vi "startTcpServer.vi"(8 "error in (no error)":errorcluster) -> (0 "error out":errorcluster, 2 "TcpServer out":refnum<class "TcpServer.lvclass">, 3 "UserEvents":T1)   [LabVIEW 2018]
doc: "Start the TCP server."
uses:
  src/TcpServer/TcpServer.lvclass
  src/TcpServerBase/typedef/connStatusCluster.ctl
  src/TcpServer/configServerTypeDef.ctl
  src/TcpServerTel/typedef/enqueueOptionsTypeDef.ctl
  src/FactoryTcpServer/FactoryTcpServer.lvclass
  src/TcpServer/runServer.vi
  src/TcpServerTel/TcpServerTel.lvclass
  src/TcpServerBase/TcpServerBase.lvclass
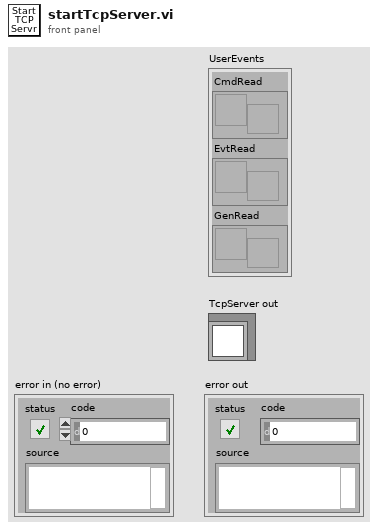
[diagram p1: front panel]
types:
  T1 = cluster{"CmdRead":refnum<user-event>, "EvtRead":refnum<user-event>, "GenRead":refnum<user-event>}
  T2 = typedef "TcpServer.lvclass/configServerTypeDef.ctl" = cluster{"cmdServerPort":u16, "telServerPort":u16, "timeoutServerInMs":i32, "serverBytesToRead":i32, "maxSizeQueueTcpClientFromDds":i32, "EnqueueOptions":T3, "timeoutQueueTcpClientFromDds (ms)":i32, "maxSizeQueueTcpClient":i32, "timeoutInMs":i32}
  T3 = typedef "TcpServerTel.lvclass/enqueueOptionsTypeDef.ctl" = enum16{"lossy enqueue", "normal enqueue"}
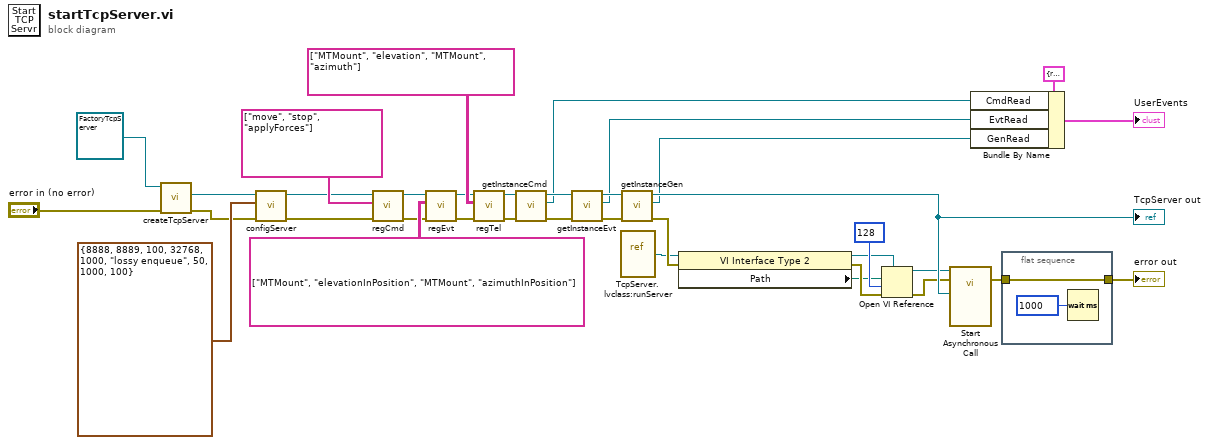
[diagram p0: block diagram]
diagram:
  n1 = call "createTcpServer.vi"("error in (no error)"="error in (no error)", "FactoryTcpServer in"=refnum<class "FactoryTcpServer.lvclass"> refnum) -> ("error out"=w3:errorcluster, "TcpServer out"=w4:refnum<class "TcpServer.lvclass">)  [unwired: 7 in, 1 out]
  n2 = call "configServer.vi"("error in (no error)"=w3, "ServerConfiguration"=T2 {"cmdServerPort"=8888, "telServerPort"=8889, "timeoutServerInMs"=100, "serverBytesToRead"=32768, "maxSizeQueueTcpClientFromDds"=1000, "EnqueueOptions"=enum."lossy enqueue", "timeoutQueueTcpClientFromDds (ms)"=50, "maxSizeQueueTcpClient"=1000, "timeoutInMs"=100}, "tcpServer in"=w4) -> ("error out"=w32:errorcluster, "tcpServer out"=w13:refnum<class "TcpServer.lvclass">)  [unwired: 7 in]
  n3 = call "regCmd.vi"("error in (no error)"=w32, "cmdReg"=string[] ["move", "stop", "applyForces"], "tcpServer in"=w13) -> ("error out"=w12:errorcluster, "tcpServer out"=w25:refnum<class "TcpServer.lvclass">)  [unwired: 7 in]
  n4 = call "regEvt.vi"("error in (no error)"=w12, "evtReg"=string[][] [["MTMount", "elevationInPosition"], ["MTMount", "azimuthInPosition"]], "tcpServer in"=w25) -> ("error out"=w24:errorcluster, "tcpServer out"=w29:refnum<class "TcpServer.lvclass">)  [unwired: 7 in]
  n5 = call "regTel.vi"("error in (no error)"=w24, "telReg"=string[][] [["MTMount", "elevation"], ["MTMount", "azimuth"]] ("regTel"), "tcpServer in"=w29) -> ("error out"=w28:errorcluster, "tcpServer out"=w30:refnum<class "TcpServer.lvclass">)  [unwired: 7 in]
  n6 = call "getInstanceCmd.vi"("error in (no error)"=w28, "tcpServer in"=w30) -> ("error out"=w14:errorcluster, "CmdRead"=w10:refnum<user-event>, "tcpServer out"=w16:refnum<class "TcpServer.lvclass">)  [unwired: 7 in]
  n7 = call "getInstanceEvt.vi"("error in (no error)"=w14, "tcpServer in"=w16) -> ("error out"=w15:errorcluster, "EvtRead"=w9:refnum<user-event>, "tcpServer out"=w27:refnum<class "TcpServer.lvclass">)  [unwired: 7 in]
  n8 = vi-ref "TcpServer.lvclass:runServer.vi"() -> (w17:refnum<vi>)
  n9 = call "getInstanceGen.vi"("error in (no error)"=w15, "tcpServer in"=w27) -> ("error out"=w26:errorcluster, "GenRead"=w8:refnum<user-event>, "tcpServer out"=w36:refnum<class "TcpServer.lvclass">)  [unwired: 7 in]
  "TcpServer out" <- w36
  n10 = property class="VI Interface Type 2"(reference=w17, error in=w26) -> (reference out=w19:refnum<vi>, error out=w22:errorcluster, "Path"=w18:path)
  n11 = Open VI Reference(type specifier VI Refnum (for type only)=w19, vi path=w18, options=128, error in (no error)=w22) -> (vi reference=w21:refnum<vi>, error out=w23:errorcluster)  [unwired: 2 in]
  n12 = call-by-ref "Start Asynchronous Call"(reference=w21, error in=w23, "TcpServer in"=w36) -> (error out=w5:errorcluster)  [unwired: 9 in, 3 out]
  n13 = Bundle By Name(cluster=T1 {"CmdRead"=refnum, "EvtRead"=refnum, "GenRead"=refnum}, "CmdRead"=w10, "EvtRead"=w9, "GenRead"=w8) -> (→"UserEvents":T1)
  n14 = flat-sequence {
    tunnel: [w37] -> w6
    tunnel: w5 -> [w37]
    frame #0 {
      n15 = Wait (ms)(milliseconds to wait=u32 1000) -> ()  [unwired: 1 out]
    }
  }
  "error out" <- w6
